vi "Prussure_Tester_V2.vi"() -> ()   [LabVIEW 2015]
uses:
  <vilib>/Waveform/WDTOps.llb/WDT Append Waveforms DBL.vi
panel:
  in  "Filename":path=path "C:/Users/Mechanical/Desktop/Loard Star - Strain gauge/Load star test/test1.lvm"
  in  "Pressure/Volt Gain (Typ. 5)":dbl
  out "Original Signal":waveform(dbl)(graph)
  out "Pressure Value":waveform(dbl)(graph)
  in  "number of samples":i32=10
  in  "rate":dbl
  in  "stop":bool
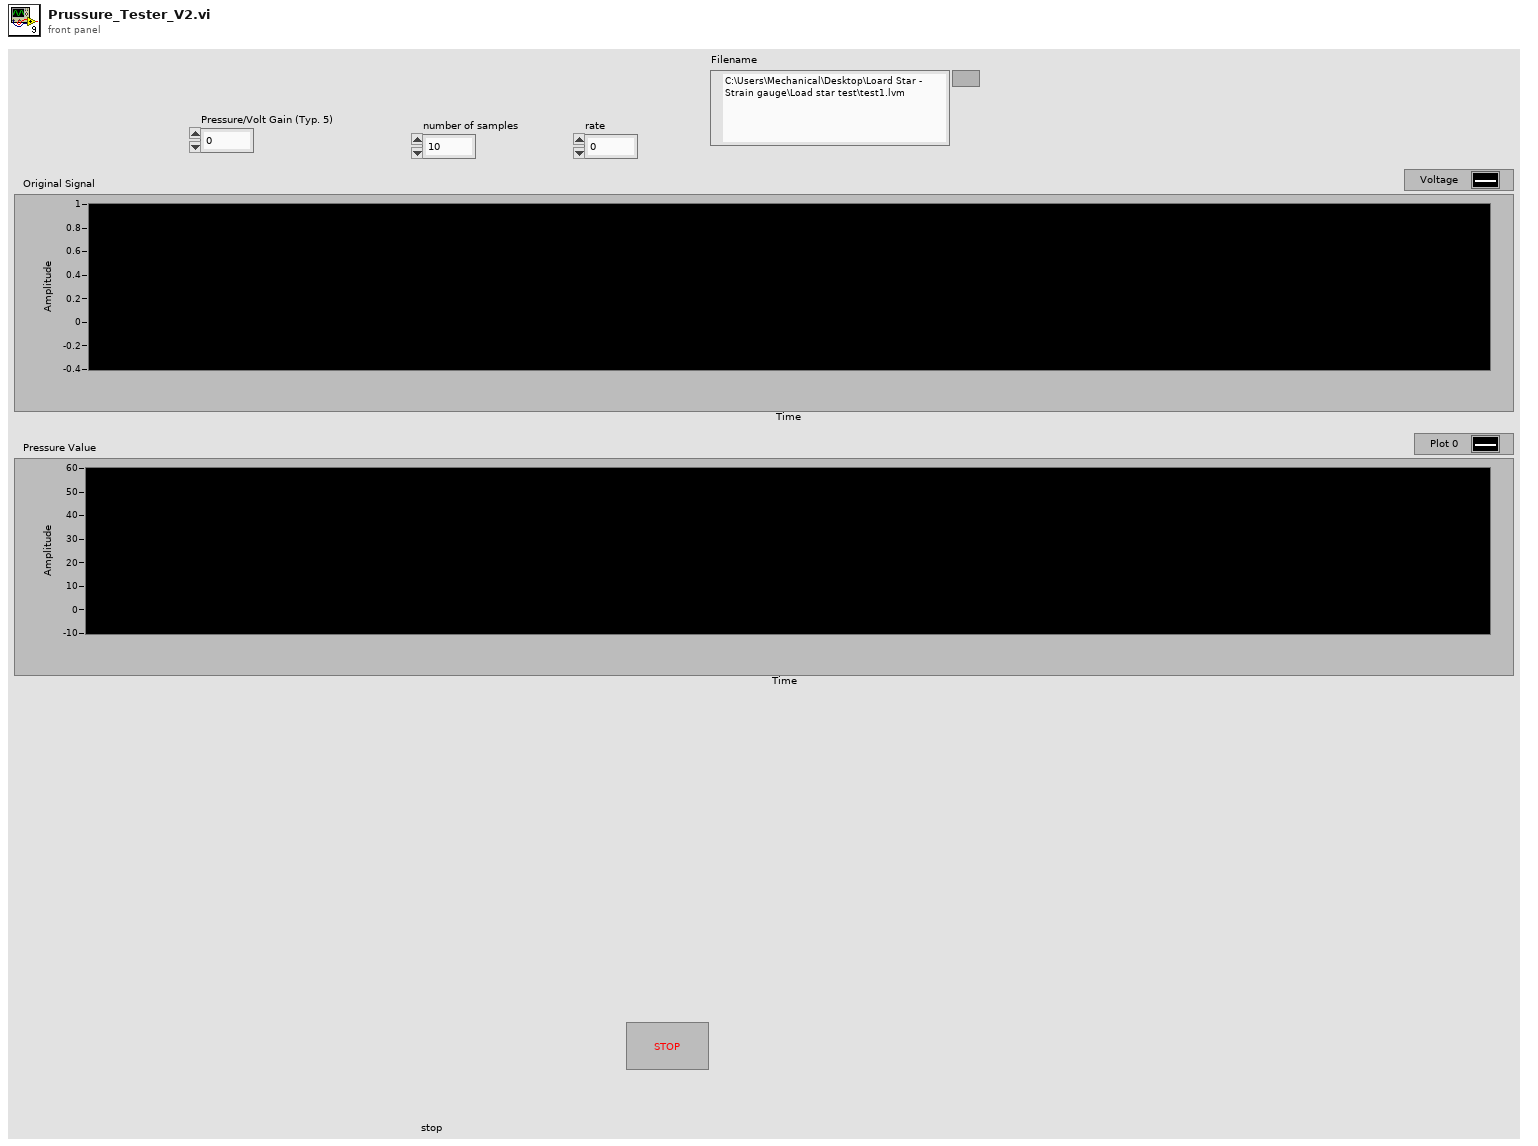
[diagram p1: front panel]
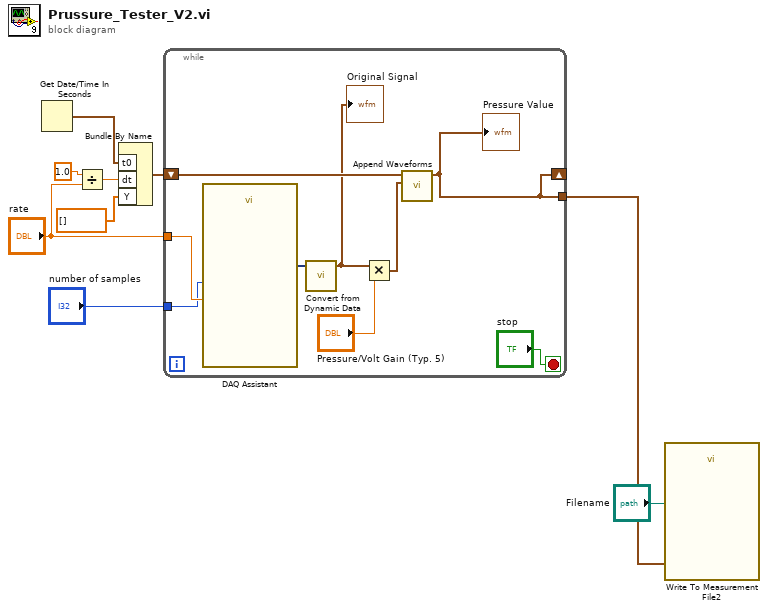
[diagram p0: block diagram]
diagram:
  n1 = Get Date/Time In Seconds() -> (seconds since 1Jan1904=w8:timestamp)
  n2 = Divide(x=1.0, y="rate") -> (x/y=w6:dbl)
  n3 = Bundle By Name("t0"=w8, "dt"=w6, "Y"=dbl[] []) -> (w9:waveform(dbl))  [unwired: 1 in]
  n4 = while {
    shift-right: [w13] -> _
    shift-left: w9 -> [w15]
    tunnel: "rate" -> [w17]
    tunnel: "number of samples" -> [w16]
    tunnel: [w13] -> w2
    stop <- "stop" stop-if-true
    n5 = call "DAQ Assistant"("rate"=w17, "number of samples"=w16) -> ("data"=w14:dynamicdata)  [unwired: 15 in, 2 out]
    n6 = call "Convert from Dynamic Data"("Dynamic Data Type"=w14) -> ("Waveform"=w11:waveform(dbl))  [unwired: 3 in]
    "Original Signal" <- w11
    n7 = Multiply(x=w11, y="Pressure/Volt Gain (Typ. 5)") -> (x*y=w12:waveform(dbl))
    n8 = call-poly <vilib>:"Append Waveforms.vi"("waveform B"=w12, "waveform A"=w15) -> ("waveform out"=w13:waveform(dbl))  [unwired: 8 in, 1 out]
    "Pressure Value" <- w13
  }
  n9 = call "Write To Measurement File2"("Signals"=w2, "Filename"="Filename") -> ()  [unwired: 15 in, 3 out]
